vi "broadcast ROI data.vi"(8 "error in (no error)":errorcluster, 11 "Camera Process in":refnum<class "Camera Process.lvclass">) -> (0 "error out":errorcluster, 3 "Camera Process in 2":refnum<class "Camera Process.lvclass">)   [LabVIEW 2022 SP3, in "Cam Process.lvlib" / "Camera Process.lvclass"]
uses:
  Camera Process.lvclass
  Camera Process.lvclass/Camera Process.ctl
  Camera Data/Camera Data.lvclass/Camera Data.ctl
  Camera Data/Read ROI.vi
  Camera Data/Read Events.vi
  <vilib>/vision/NI_Vision_Development_Module.lvlib
  Camera Data/Camera Data.lvclass
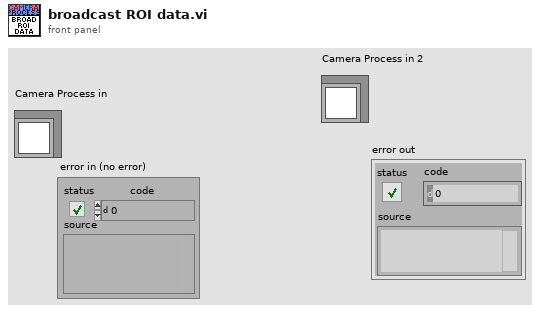
[diagram p1: front panel]
types:
  T1 = typedef "IMAQ Image.ctl" = refnum<image>
  T2 = cluster{"Global Rectangle":i32[], "Contours":cluster{"Contour Type":u32, "ROI Type":u32, "Points":i32[]}[]}
  T3 = typedef "Camera Data.lvclass/events.ctl" = cluster{"Image":refnum<user-event>, "Min Value":refnum<user-event>, "Max Value":refnum<user-event>, "Mean Value":refnum<user-event>, "Standard  Variation":refnum<user-event>}
  T4 = cluster{"histogram":u32[], "Minimal Value":sgl, "Maximal Value":sgl, "Starting Value":sgl, "Interval Width":sgl, "Mean Value":sgl, "Standard  Variation":sgl, "Area (pixels)":i32}
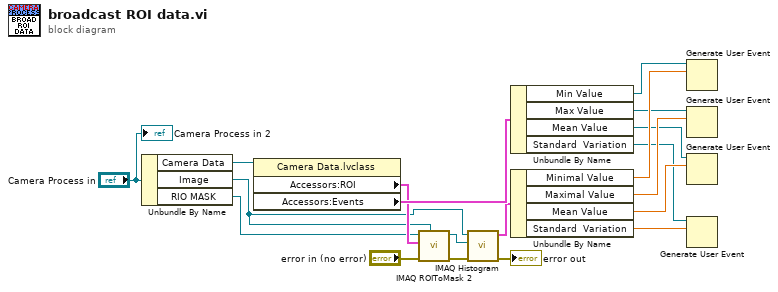
[diagram p0: block diagram]
diagram:
  n1 = Unbundle By Name("Camera Process in") -> ("Camera Data"=w7:refnum<data-value>, "Image"=w5:T1, "RIO MASK"=w4:T1)
  n2 = property class="Camera Data.lvclass"(reference=w7) -> ("Accessors:ROI"=w8:T2, "Accessors:Events"=w10:T3)  [unwired: 1 in, 2 out]
  n3 = call "IMAQ ROIToMask 2"("Image Model"=w5, "error in (no error)"="error in (no error)", "ROI Descriptor"=w8, "Image"=w4) -> ("error out"=w2:errorcluster, "Image Out"=w6:T1)  [unwired: 5 in, 1 out]
  n4 = call "IMAQ Histogram"("error in (no error)"=w2, "Image Mask"=w6, "Image"=w5) -> ("error out"=→"error out":errorcluster, "Histogram Report"=w9:T4)  [unwired: 7 in]
  n5 = Unbundle By Name(w10) -> ("Min Value"=w11:refnum<user-event>, "Max Value"=w12:refnum<user-event>, "Mean Value"=w13:refnum<user-event>, "Standard  Variation"=w14:refnum<user-event>)
  n6 = Unbundle By Name(w9) -> ("Minimal Value"=w15:sgl, "Maximal Value"=w16:sgl, "Mean Value"=w17:sgl, "Standard  Variation"=w18:sgl)
  n7 = Generate User Event(user event=w11, event data cluster=w15) -> ()  [unwired: 2 in, 2 out]
  n8 = Generate User Event(user event=w12, event data cluster=w16) -> ()  [unwired: 2 in, 2 out]
  n9 = Generate User Event(user event=w13, event data cluster=w17) -> ()  [unwired: 2 in, 2 out]
  n10 = Generate User Event(user event=w14, event data cluster=w18) -> ()  [unwired: 2 in, 2 out]
  "Camera Process in 2" <- "Camera Process in"
